vi "BGK8001 Protocol.vi"(3 "字符串":string) -> (0 "timestamp":timestamp caption="时间标识", 1 "数组":dbl[](array[numeric]))   [LabVIEW 2015]
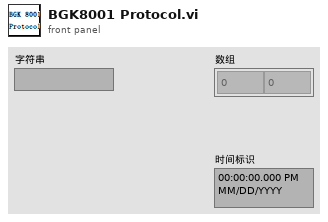
[diagram p1: front panel]
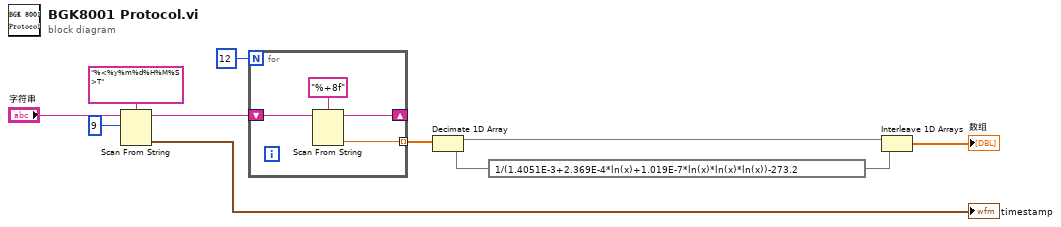
[diagram p0: block diagram]
diagram:
  n1 = Scan From String(format string="%<%y%m%d%H%M%S>T" ("格式字符串"), input string="字符串", initial scan location=u32 9 ("初始扫描位置")) -> (remaining string=w10:string, output 1=→"timestamp":timestamp)  [unwired: 2 in, 2 out]
  n2 = for {
    N: 12 -> [_]
    tunnel: [w13] -> w8 mode=indexing
    shift-right: [w12] -> _
    shift-left: w10 -> [w15]
    n3 = Scan From String(format string="%+8f" ("格式字符串"), input string=w15) -> (remaining string=w12:string, output 1=w13:dbl)  [unwired: 3 in, 2 out]
  }
  n4 = Decimate 1D Array(w8) -> (w5:dbl[], w6:dbl[])
  n5 = expression code="1/(1.4051E-3+2.369E-4*ln(x)+1.019E-7*ln(x)*ln(x)*ln(x))-273.2"(w6) -> (w4:dbl[])
  n6 = Interleave 1D Arrays(w5, w4) -> (→"数组":dbl[])
